vi "firstCalculationsDISS.vi"() -> ()   [LabVIEW 2020]
uses:
  <vilib>/Utility/file.llb/Read Delimited Spreadsheet (string).vi
panel:
  in  "Path 2":path
  out "Path":path
  out "v = a(deltaT)":dbl
  out "Numeric":dbl
  out "Date":string
  in  "Numeric 2":dbl
  in  "StationID":string
  out "n":dbl
  out "ZT":dbl
  in  "Seebeck Coe":dbl
  out "nCarrot":dbl
  out "delta T":dbl
  out "Temp hot":dbl
  out "Temp cold":dbl
  out "Thermal Conductivity":dbl
  in  "Thermal Resistance":dbl=2.16
  in  "Area":dbl=2.712
  in  "Thickness":dbl=0.00135
  out "ELECTRIC CONDUCTIVITY":dbl
  in  "ELECTRIC RESISTANCE":dbl=2.16
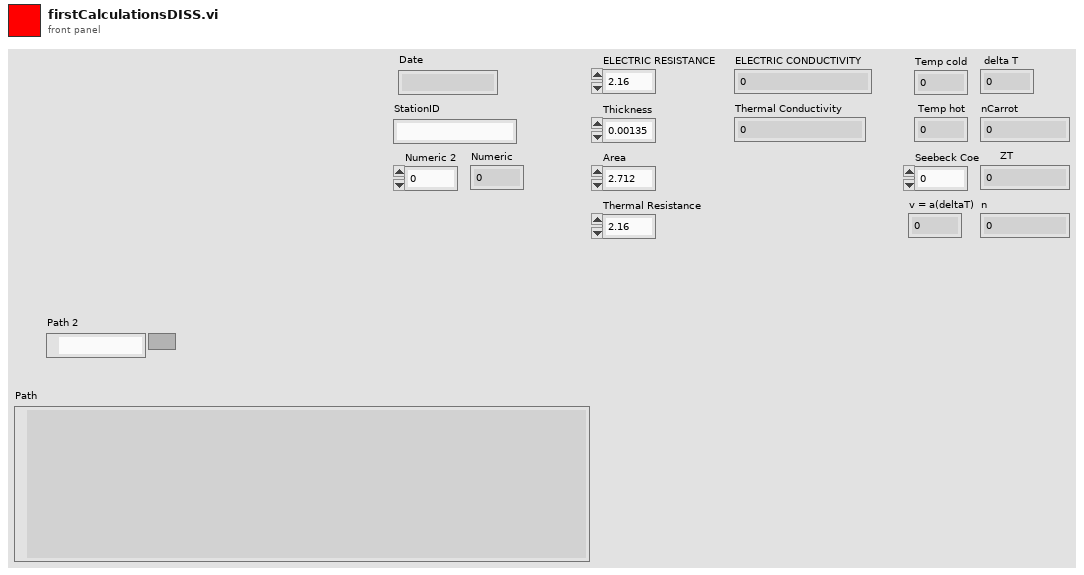
[diagram p1: front panel]
types:
  T1 = cluster{"String 2":string, "String 3":string, "String 4":string, "String 5":string, "String 6":string, "String 7":string}
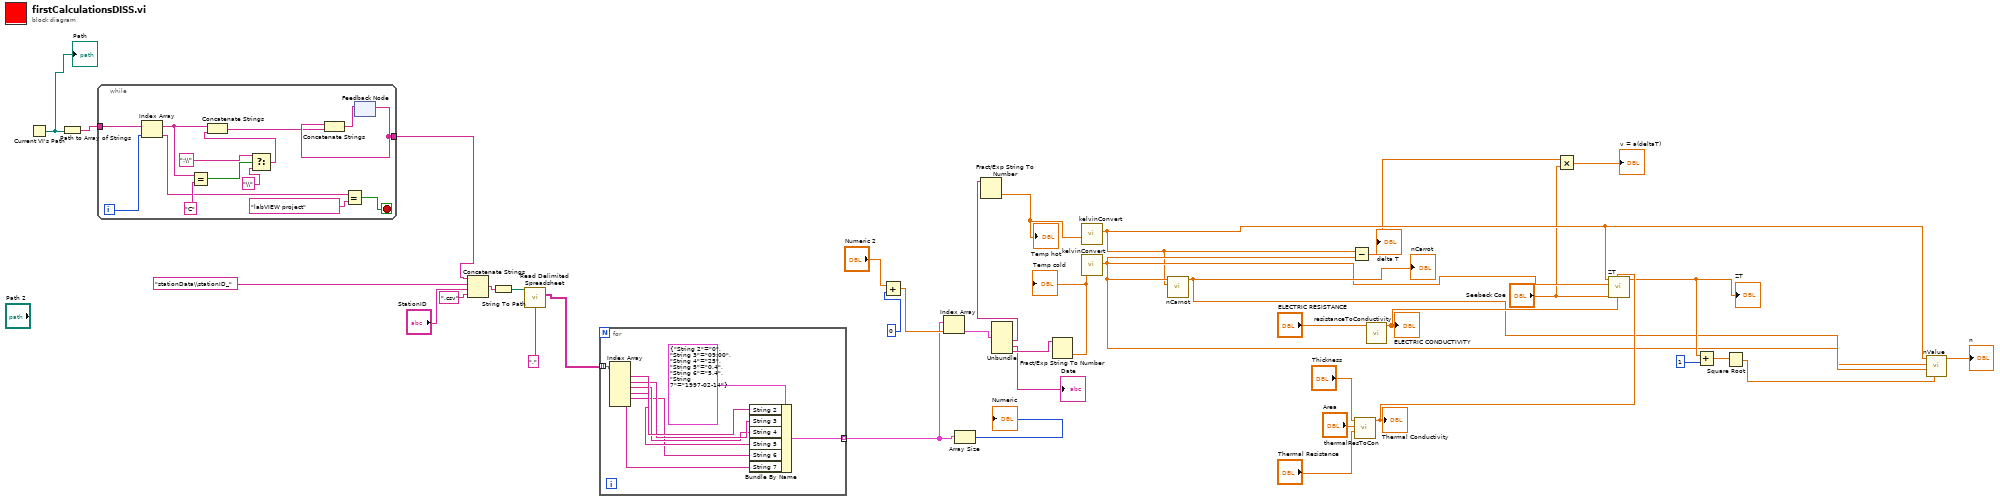
[diagram p0: block diagram]
diagram:
  n1 = Current VI's Path() -> (path=w1:path)
  "Path" <- w1
  n2 = Path to Array of Strings(0:w1) -> (2:w3:string[])  [unwired: 1 out]
  n3 = while {
    tunnel: w3 -> [w49]
    tunnel: [w40] -> w7
    i -> [w48]
    stop <- w51 stop-if-true
    n4 = Index Array(array=w49, index=w48) -> (element=w42:string)
    n5 = Equal?(x=w42, y="C") -> (x = y?=w46:bool)
    n6 = Select(t=":\\", s=w46, f="\\") -> (s? t:f=w43:string)
    n7 = Concatenate Strings(w42, w43) -> (w39:string)
    n8 = Equal?(x=w42, y="labVIEW project") -> (x = y?=w51:bool)
    n9 = feedback #1() -> (w40:string)  [unwired: 1 in]
    n10 = Concatenate Strings(w40, w39) -> (w41:string)
    n11 = feedback-in #1(w41) -> ()
  }
  n12 = Concatenate Strings(w7, "stationData\\stationID_", "StationID", ".csv") -> (w21:string)
  n13 = String To Path(string=w21) -> (path=w2:path)
  n14 = call-poly <vilib>:"Read Delimited Spreadsheet.vi"("file path (dialog if empty)"=w2, "delimiter (\\t)"="," ("delimiter (\\t)")) -> ("all rows"=w19:string[][])  [unwired: 8 in, 5 out]
  n15 = for {
    tunnel: w19 -> [w60] mode=indexing
    tunnel: [w53] -> w10 mode=indexing
    n16 = Index Array(array=w60) -> (element #1=w58:string, element #2=w57:string, element #3=w56:string, element #4=w55:string, element #5=w54:string, element #6=w52:string)  [unwired: 6 in]
    n17 = Bundle By Name(cluster=T1 {"String 2"="0", "String 3"="09:00", "String 4"="25", "String 5"="0.4", "String 6"="5.4", "String 7"="1997-02-14"} ("Cluster"), "String 2"=w58, "String 3"=w57, "String 4"=w56, "String 5"=w55, "String 6"=w54, "String 7"=w52) -> (w53:T1)
  }
  n18 = Add(x="Numeric 2", y=0 ("index")) -> (x+y=w11:dbl)
  n19 = Index Array(array=w10, index=w11) -> (element=w18:T1)
  n20 = Array Size(array=w10) -> (size(s)=→"Numeric":i32)
  n21 = Unbundle(w18) -> ("String 5"=w14:string, "String 6"=→"Date":string, "String 7"=w15:string)  [unwired: 3 out]
  n22 = Fract/Exp String To Number(string=w14) -> (number=w13:dbl)  [unwired: 3 in, 1 out]
  "Temp hot" <- w13
  n23 = Fract/Exp String To Number(string=w15) -> (number=w12:dbl)  [unwired: 3 in, 1 out]
  "Temp cold" <- w12
  n24 = call "kelvinConvert.vi"("Temp hot"=w13) -> ("Numeric"=w26:dbl)  [unwired: 2 in]
  n25 = call "kelvinConvert.vi"("Temp hot"=w12) -> ("Numeric"=w27:dbl)  [unwired: 2 in]
  n26 = call "nCarnot.vi"("Temp hot"=w26, "Numeric"=w27) -> ("nCarrot"=w28:dbl)  [unwired: 9 in]
  "nCarrot" <- w28
  n27 = Subtract(x=w26, y=w27) -> (x-y=w6:dbl)
  "delta T" <- w6
  n28 = call "thermalResToCon.vi"("Thermal Resistance"="Thermal Resistance", "Area"="Area", "Thickness"="Thickness") -> ("Thermal Conductivity"=w33:dbl)  [unwired: 8 in]
  "Thermal Conductivity" <- w33
  n29 = call "resistanceToConductivity.vi"("ELECTRIC RESISTANCE"="ELECTRIC RESISTANCE") -> ("Numeric"=w34:dbl)  [unwired: 10 in]
  "ELECTRIC CONDUCTIVITY" <- w34
  n30 = Multiply(x=w6, y="Seebeck Coe") -> (x*y=→"v = a(deltaT)":dbl)
  n31 = call "ZT.vi"("Numeric"=w34, "Thermal Conductivity"=w33, "Seebeck Coe"="Seebeck Coe", "Numeric 2"=w27, "Numeric 3"=w26) -> ("ZT"=w30:dbl)  [unwired: 6 in]
  "ZT" <- w30
  n32 = Add(x=w30, y=1) -> (x+y=w31:dbl)
  n33 = Square Root(x=w31) -> (sqrt(x)=w29:dbl)
  n34 = call "nValue.vi"("Numeric 3"=w29, "nCarrot"=w28, "Numeric 2"=w27, "Numeric"=w26) -> ("n"=→"n":dbl)  [unwired: 7 in]
